vi "Link Bus A Parameters.vi"(8 "error in (no error)":errorcluster, 11 "Bus Monitor in":refnum<class "Bus Monitor.lvclass">) -> (0 "error out":errorcluster, 3 "Bus Monitor out":refnum<class "Bus Monitor.lvclass">)   [LabVIEW 2020, in "BCI-1553 API.lvlib" / "Bus Monitor.lvclass"]
doc: "Creates a Bus Monitor-Only table of all the filters that will be operating on Bus A. This table uses command words as keys where the Word Count and Mode Code has been masked to 1F. This is used for quickly performing lookups on the current state of the monitored parameters identified in the filter. When a filter command word is not found, it remains with an unmodified value."
uses:
  Bus Monitor.lvclass
  Bus Monitor.lvclass/Bus Monitor.ctl
  Dependencies/Registry/Registry.lvclass/Registry.ctl
  Filters/Filter/Filter.lvclass
  <vilib>/Utility/error.llb/Clear Errors.vi
  Dependencies/Registry/Registry.lvclass
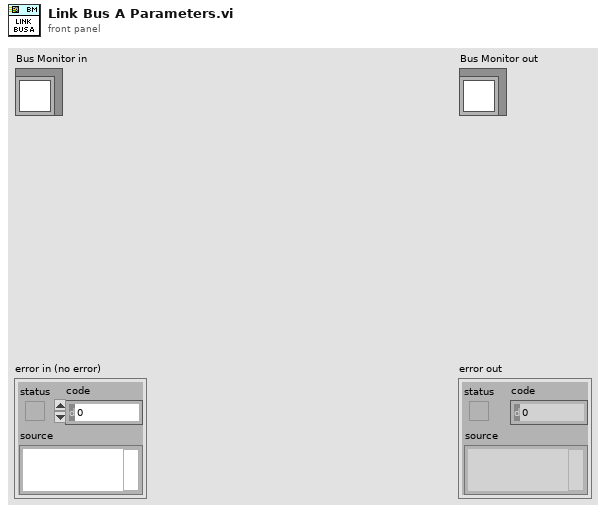
[diagram p1: front panel]
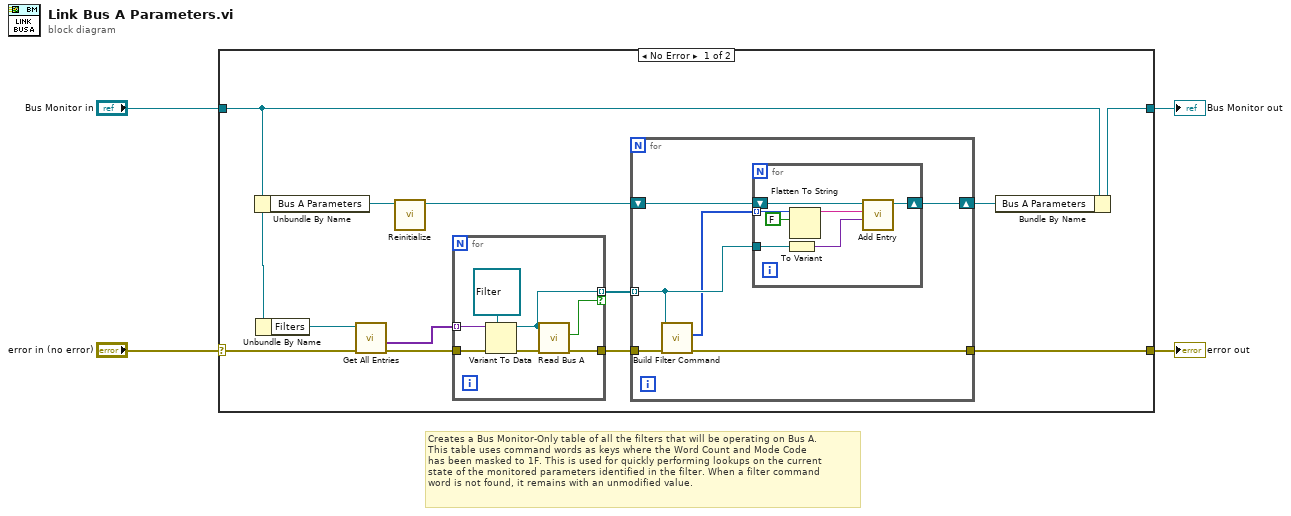
[diagram p0: block diagram]
diagram:
  # "Creates a Bus Monitor-Only table of all the filters that will be operating on Bus A.\nThis table uses command words as keys where the Word Count and Mode Code\nhas been masked to 1F. This is used for quickly performing lookups on the current\nstate of the monitored parameters identified in the filter. When a filter command\nword is not found, it remains with an unmodified value."
  n1 = case shown="No Error" "error in (no error)" {
    selector: "error in (no error)" -> [w14 w38]
    tunnel: [w10 w38] -> w3
    tunnel: [w5 w37] -> w1
    tunnel: "Bus Monitor in" -> [w6 w37]
    frame No Error {
      n2 = Unbundle By Name(w6) -> ("Bus A Parameters"=w16:refnum<class "Registry.lvclass">)
      n3 = Unbundle By Name(w6) -> ("Filters"=w15:refnum<class "Registry.lvclass">)
      n4 = call "Get All Entries.vi"("error in (no error)"=w14, "Registry in"=w15) -> ("error out"=w13:errorcluster, "Values"=w12:variant[])  [unwired: 7 in, 1 out]
      n5 = call "Reinitialize.vi"("Registry in"=w16) -> ("Registry out"=w8:refnum<class "Registry.lvclass">)  [unwired: 9 in, 1 out]
      n6 = for {
        tunnel: w12 -> [w35] mode=indexing
        tunnel: w13 -> [w33]
        tunnel: [w36] -> w11
        tunnel: [w31] -> w9 mode=indexing if=w30
        n7 = Variant To Data(error in=w33, type=refnum<class "Filter.lvclass"> refnum ("SLSC 1553 API.lvlib:Filter.lvclass"), Variant=w35) -> (data=w31:refnum<class "Filter.lvclass">, error out=w32:errorcluster)
        n8 = call-dynamic "Read Bus A.vi"("error in (no error)"=w32, "Filter in"=w31) -> ("error out"=w36:errorcluster, "Bus A?"=w30:bool)  [unwired: 7 in, 1 out]
      }
      n9 = for {
        tunnel: w11 -> [w22]
        tunnel: [w21] -> w10
        tunnel: w9 -> [w19] mode=indexing
        shift-right: [w18] -> w7
        shift-left: w8 -> [w20]
        n10 = call-dynamic "Build Filter Command.vi"("error in (no error)"=w22, "Filter in"=w19) -> ("error out"=w21:errorcluster, "Command Words"=w17:u16[])  [unwired: 8 in]
        n11 = for {
          shift-right: [w25] -> w18
          shift-left: w20 -> [w26]
          tunnel: w17 -> [w29] mode=indexing
          tunnel: w19 -> [w27]
          n12 = To Variant(anything=w27) -> (Variant=w24:variant)
          n13 = Flatten To String(anything=w29, prepend array or string size? (T)=FALSE) -> (data string=w23:string)  [unwired: 2 in, 2 out]
          n14 = call "Add Entry.vi"("Value"=w24, "Key"=w23, "Registry in"=w26) -> ("Registry out"=w25:refnum<class "Registry.lvclass">)  [unwired: 6 in, 2 out]
        }
      }
      n15 = Bundle By Name(cluster=w6, "Bus A Parameters"=w7) -> (w5:refnum<class "Bus Monitor.lvclass">)
    }
    frame Error {
    }
  }
  "error out" <- w3
  "Bus Monitor out" <- w1
